vi "PPS_Aquire.vi"(2 "error in":errorcluster, 3 "fpga ref":refnum<k20>) -> (0 "error out":errorcluster, 1 "fpga ref return":refnum<k20>)   [LabVIEW 2015]
uses:
  PPS_Global_Var.vi
  <vilib>/Utility/error.llb/Error Cluster From Error Code.vi
  <vilib>/rvi/errors/niLvFpgaAdjustHostInterfaceError.vi
  Supporting Files/test_sup.vi
  <vilib>/rvi/interface/nirviReadWriteControl/nirviReadWriteControl.xnode
  <vilib>/rvi/interface/nirviMethod/nirviMethod.xnode
  NiFpgaLv.dll
  <vilib>/rvi/interface/Simulation/niFpgaSimulationCallBeginRW.vi
  <vilib>/FPGAPlugInAG/Dynamic/niLvFpga_ReadFifo_Dynamic.vi
  <vilib>/rvi/errors/niLvFpgaMergeErrorWithErrorCode.vi
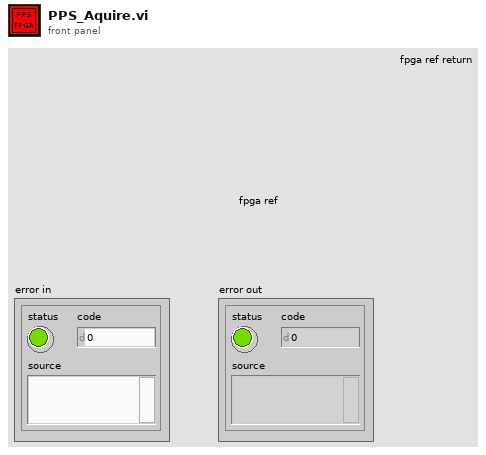
[diagram p1: front panel]
types:
  T1 = cluster{"Data[0]":u64, "Data[1]":u64, "Data[2]":u64, "Data[3]":u64, "Data[4]":u64, "Data[5]":u64, "Data[6]":u64, "Data[7]":u64, "Data[8]":u64}
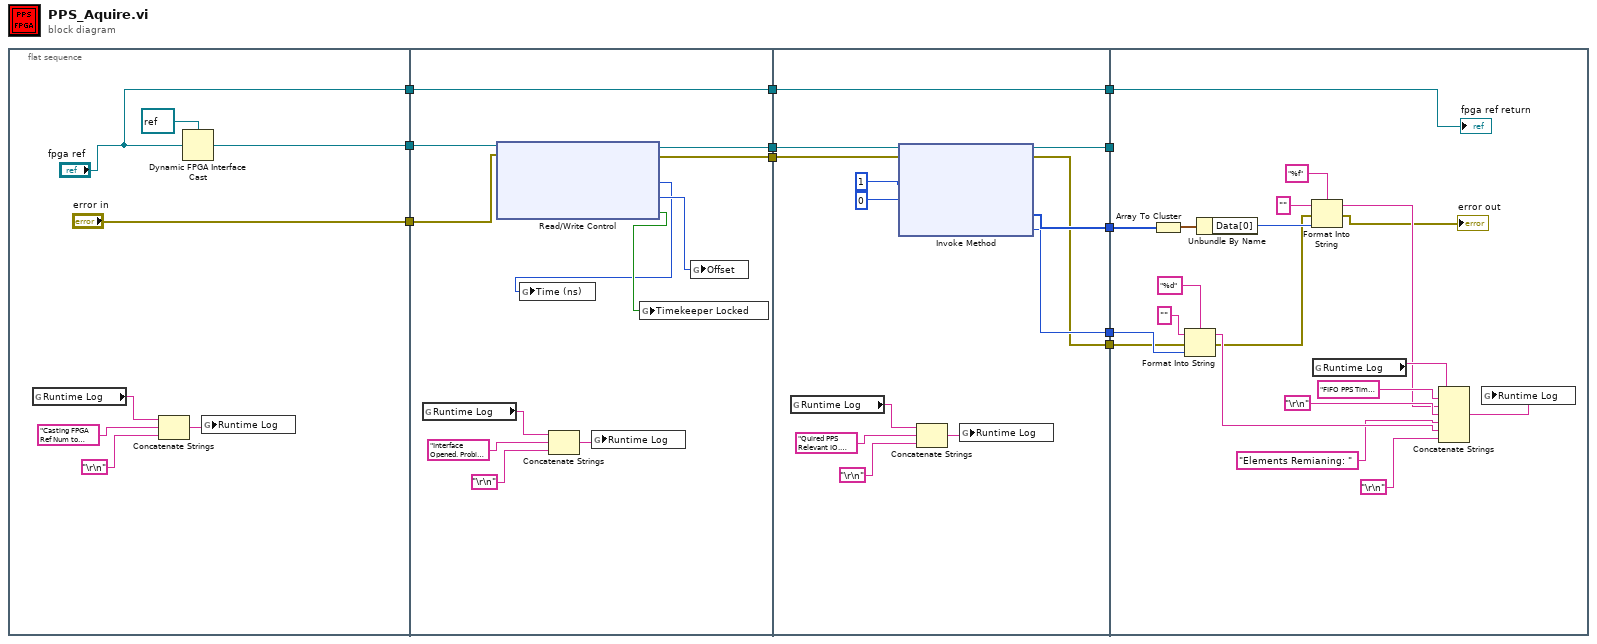
[diagram p0: block diagram]
diagram:
  n1 = flat-sequence {
    tunnel: [w14] -> w11
    tunnel: ["error in"] -> w4
    tunnel: ["fpga ref"] -> w3
    tunnel: w11 -> [w27]
    tunnel: [w26] -> w10
    tunnel: [w25] -> w5
    tunnel: w4 -> [w24]
    tunnel: w3 -> [w23]
    tunnel: [w23] -> w2
    tunnel: w10 -> [w40]
    tunnel: [w37] -> w9
    tunnel: [w36] -> w8
    tunnel: [w35] -> w7
    tunnel: [w34] -> w6
    tunnel: w5 -> [w33]
    tunnel: w2 -> [w32]
    tunnel: [w32] -> w1
    tunnel: w9 -> [w57]
    tunnel: w8 -> [w54]
    tunnel: w7 -> [_]
    tunnel: w6 -> [w46]
    tunnel: w1 -> [w45]
    frame #0 {
      n2 = global read "PPS_Global_Var.vi" "Runtime Log"() -> (w17:string)
      n3 = Concatenate Strings(w17, "Casting FPGA Ref Num to Type", "\r\n") -> (w18:string)
      n4 = Dynamic FPGA Interface Cast(Session In=refnum<k20> refnum ("FPGA Interface"), Type="fpga ref") -> (Session Out=w14:refnum<k20>)
      n5 = global write "PPS_Global_Var.vi" "Runtime Log"(w18) -> ()
    }
    frame #1 {
      n6 = global read "PPS_Global_Var.vi" "Runtime Log"() -> (w30:string)
      n7 = xnode "Read/Write Control"("FPGA VI Reference In"=w27, "error in"=w24) -> ("FPGA VI Reference Out"=w26:refnum<k20>, "error out"=w25:errorcluster, "FPGA Timekeeper time (ns)"=w20:u64, "offset from time reference"=w22:i32, "FPGA Timekeeper locked"=w21:bool)  [unwired: 1 out]
      n8 = global write "test_sup.vi" "Time (ns)"(w20) -> ()
      n9 = Concatenate Strings(w30, "Interface Opened. Probing IO Registers.", "\r\n") -> (w31:string)
      n10 = global write "PPS_Global_Var.vi" "Runtime Log"(w31) -> ()
      n11 = global write "test_sup.vi" "Timekeeper Locked"(w21) -> ()
      n12 = global write "test_sup.vi" "Offset"(w22) -> ()
    }
    frame #2 {
      n13 = global read "PPS_Global_Var.vi" "Runtime Log"() -> (w43:string)
      n14 = xnode "Invoke Method"("FPGA VI Reference In"=w40, "error in"=w33, "Number of Elements"=1, "Timeout (ms)"=0) -> ("FPGA VI Reference Out"=w35:refnum<k20>, "error out"=w34:errorcluster, "Data"=w37:u64[], "Elements Remaining"=w36:u32)
      n15 = Concatenate Strings(w43, "Quired PPS Relevant IO. Finding FIFO-DMA and Invoking Timestamp method. ", "\r\n") -> (w44:string)
      n16 = global write "PPS_Global_Var.vi" "Runtime Log"(w44) -> ()
    }
    frame #3 {
      n17 = Array To Cluster(array=w57) -> (cluster=w56:T1)
      n18 = Format Into String(format string="%d", initial string="", error in=w46, w54) -> (resulting string=w51:string, error out=w48:errorcluster)
      n19 = Unbundle By Name(w56) -> ("Data[0]"=w55:u64)
      n20 = Format Into String(format string="%f", initial string="", error in=w48, w55) -> (resulting string=w59:string, error out=→"error out":errorcluster)
      n21 = global read "PPS_Global_Var.vi" "Runtime Log"() -> (w63:string)
      n22 = Concatenate Strings(w63, "FIFO PPS Time stamp:", w59, "\r\n", "Elements Remianing: ", w51, "\r\n") -> (w64:string)
      n23 = global write "PPS_Global_Var.vi" "Runtime Log"(w64) -> ()
      "fpga ref return" <- w45
    }
  }
